vi "Clean local SV.vi"(8 "error in (no error)":errorcluster) -> (0 "error out":errorcluster)   [LabVIEW 2020, in "TALOS.lvlib" / "Guardian.lvlib" / "Guardian.lvclass"]
doc: "This VI just removes, at startup, all the possible remnants processes on the Shared Variable Engine."
uses:
  Guardian.lvclass
  Guardian.lvclass/Guardian.ctl
  <vilib>/lvdsc/NI_DSC.lvlib
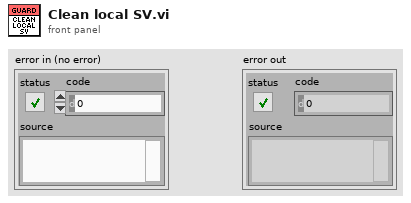
[diagram p1: front panel]
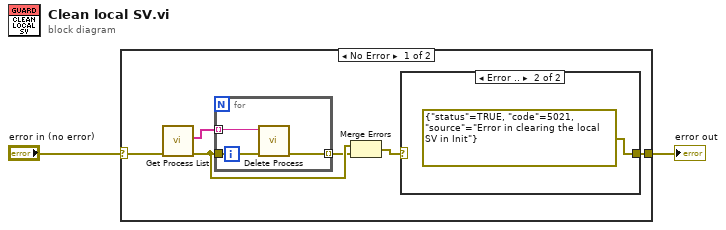
[diagram p0: block diagram]
diagram:
  n1 = case shown="No Error" "error in (no error)" {
    selector: "error in (no error)" -> [w7 w14]
    tunnel: [w3 w14] -> w1
    frame No Error {
      n2 = call <vilib>:"Get Process List.vi"("error in (no error)"=w7) -> ("error out"=w8:errorcluster, "processes"=w6:string[])  [unwired: 9 in]
      n3 = for {
        tunnel: w6 -> [w13] mode=indexing
        tunnel: w8 -> [w12]
        tunnel: [w11] -> w5 mode=indexing
        n4 = call <vilib>:"Delete Process.vi"("error in (no error)"=w12, "process name"=w13) -> ("error out"=w11:errorcluster)  [unwired: 9 in]
      }
      n5 = Merge Errors(w8, w5) -> (w4:errorcluster)
      n6 = case shown="Error .." w4 {
        selector: w4 -> [w9 _]
        tunnel: [w9 errorcluster {"status"=TRUE, "code"=5021, "source"="Error in clearing the local SV in Init"} ("error IO")] -> w3
        frame No Error {
        }
        frame Error {
        }
      }
    }
    frame Error {
    }
  }
  "error out" <- w1
